vi "Load and Execute Tests Process.vi"(0 "Operation":enum16{"Load", "Run Test", "Run All Tests"}(ring), 1 "Test Project":path, 3 "API_TextTestRunner":refnum<class>, 5 "TestTag Argument":string, 7 "Test Hierarchy Tree ref":refnum<vi>, 9 "TextStream":refnum<queue>, 11 "error in":errorcluster, 12 "TestStatusEvents":T1, 13 "AbortEvent":refnum<user-event>) -> (6 "Tree Methods":i32, 15 "error out":errorcluster)   [LabVIEW 2011, in "GraphicalTestRunner.lvlib"]
uses:
  GraphicalTestRunner.lvlib
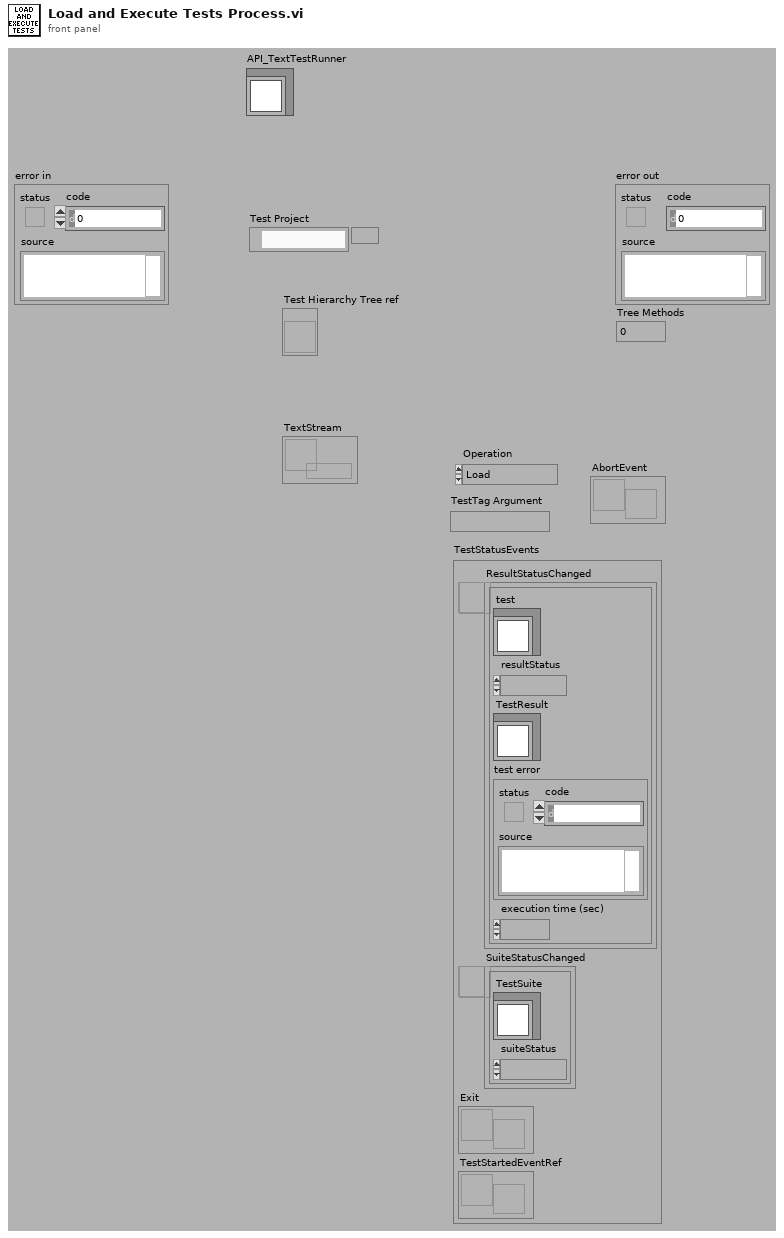
[diagram p1: front panel]
types:
  T1 = cluster{"ResultStatusChanged":refnum<user-event>, "SuiteStatusChanged":refnum<user-event>, "Exit":refnum<user-event>, "TestStartedEventRef":refnum<user-event>}
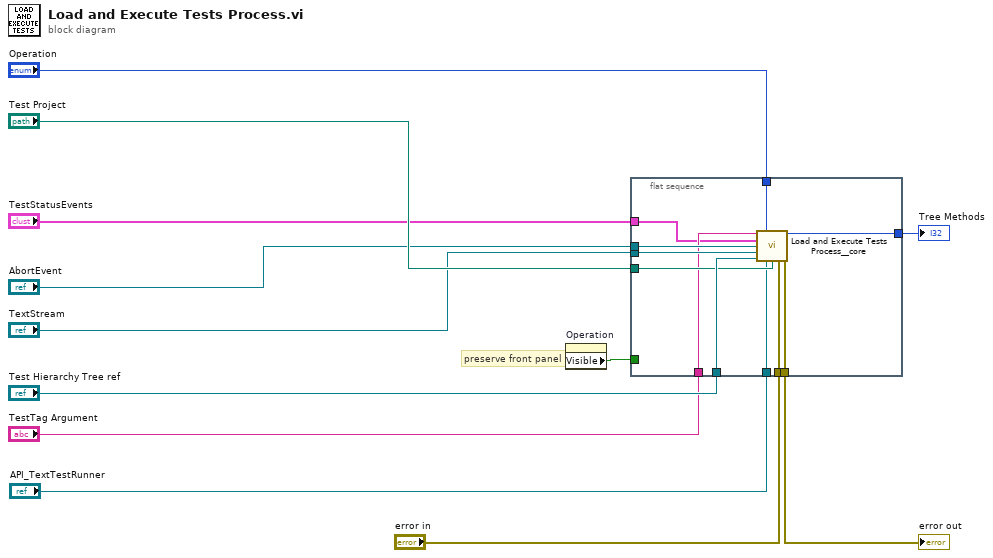
[diagram p0: block diagram]
diagram:
  # "preserve front panel"
  n1 = property on="Operation" class="Enum (strict)"() -> ("Visible"=w3:bool)  [unwired: 2 in, 2 out]
  n2 = flat-sequence {
    tunnel: "Test Hierarchy Tree ref" -> [w23]
    tunnel: "Test Project" -> [w22]
    tunnel: "error in" -> [w21]
    tunnel: "TextStream" -> [w20]
    tunnel: "Operation" -> [w19]
    tunnel: "TestTag Argument" -> [w15]
    tunnel: "AbortEvent" -> [w18]
    tunnel: "API_TextTestRunner" -> [w17]
    tunnel: [w16] -> w4
    tunnel: w3 -> [_]
    tunnel: "TestStatusEvents" -> [w14]
    tunnel: [w13] -> w1
    frame #0 {
      n3 = call "Load and Execute Tests Process__core.vi"("TestTag Argument"=w15, "Operation"=w19, "TestStatusEvents"=w14, "AbortEvent"=w18, "TextStream"=w20, "Test Hierarchy Tree ref"=w23, "API_TextTestRunner"=w17, "Test Project"=w22, "error in"=w21) -> ("Tree Methods"=w16:i32, "error out"=w13:errorcluster)  [unwired: 5 in]
    }
  }
  "error out" <- w1
  "Tree Methods" <- w4
